vi "UI - Initiate Connection_second.vi"(8 "error in (no error)":errorcluster, 10 "Controller Address":string, 11 "Message Queue":refnum<queue>) -> (0 "error out":errorcluster, 1 "Connected?":bool)   [LabVIEW 2017]
uses:
  Message Queue/Message Cluster.ctl
  controls/FPGA State.ctl
  controls/CPU Loads.ctl
  <vilib>/vision/Image Controls.llb/IMAQ Image.ctl
  Globals/Global - Configuration Options.vi
  Globals/Global - UI Stream and Variable Connections.vi
  Message Queue/Message Queue.lvlib
panel:
  out "RT Stream Name":string="FanControlSampleProject_Command Stream from RT"
  out "UI Stream Name":string="FanControlSampleProject_Command Stream from UI"
  out "error out 4":errorcluster
  out "error out 3":errorcluster
  out "error out 2":errorcluster
  out "tag acc":refnum<k21>
  out "Tag acc":refnum<k21>
  out "Variable Name Control/Indicator 2":refnum<k21>
  out "Variable Name Control/Indicator":refnum<k21>
  out "resulting string 2":string
  out "reader name":string="UI Reader"
  out "writer name":string="UI Writer"
  out "resulting string":string
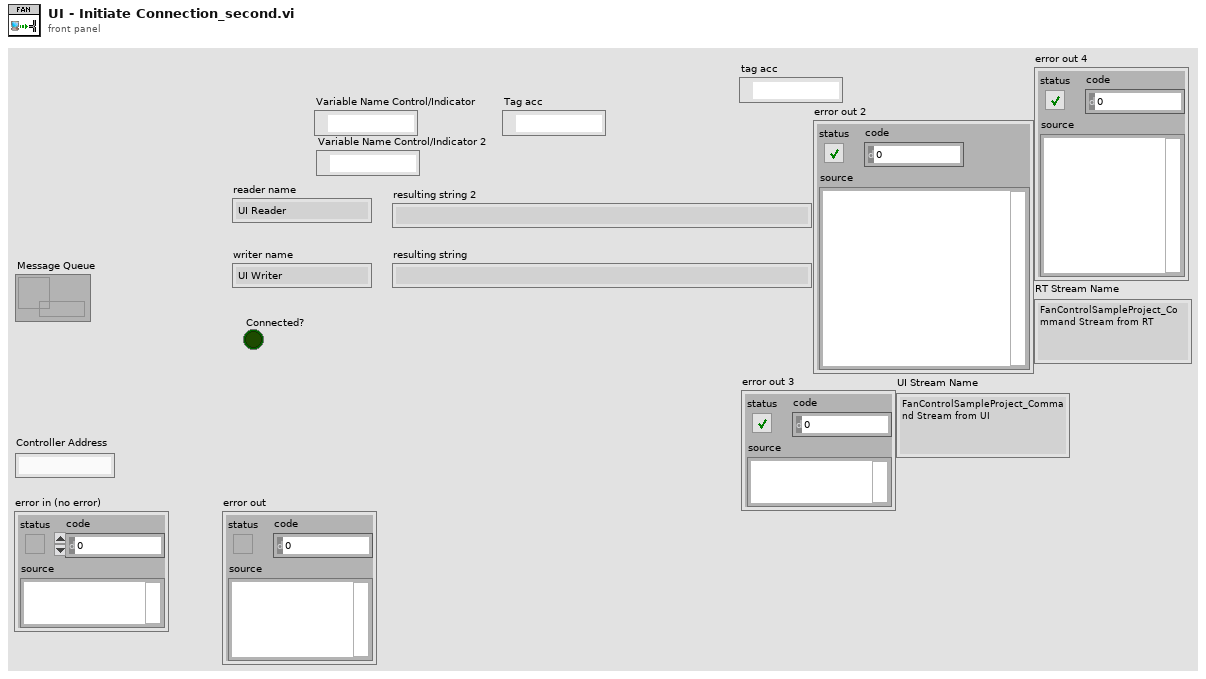
[diagram p1: front panel]
types:
  T1 = typedef "IMAQ Image.ctl" = refnum<image>
  T2 = typedef "CPU Loads.ctl" = cluster{"Total (%)":dbl, "Time Critical (%)":dbl, "Timed Structures (%)":dbl, "High (%)":dbl, "Above Normal (%)":dbl, "Normal (%)":dbl, "Background (%)":dbl, "Idle (%)":dbl, "ISR (%)":dbl}[]
  T3 = typedef "FPGA State.ctl" = enum16{"Safe State", "Control (PID)"}
  T4 = typedef "Message Queue.lvlib/Message Cluster.ctl" = cluster{"Message":string, "Message Data":variant}
  T5 = cluster{"Actual PID Loop Period":refnum<k21>, "DMA FIFO Overflow?":refnum<k21>, "CPU Usage":refnum<k21>, "Free or Contiguous Memory":refnum<k21>, "Current FPGA State":refnum<k21>, "Acceleration (grms)":refnum<k21>, "Acceleration Waveform":refnum<k21>, "Chatter":refnum<k21>, "tag acc":refnum<k21>, "tag video":refnum<k21>, "images":refnum<k21>}
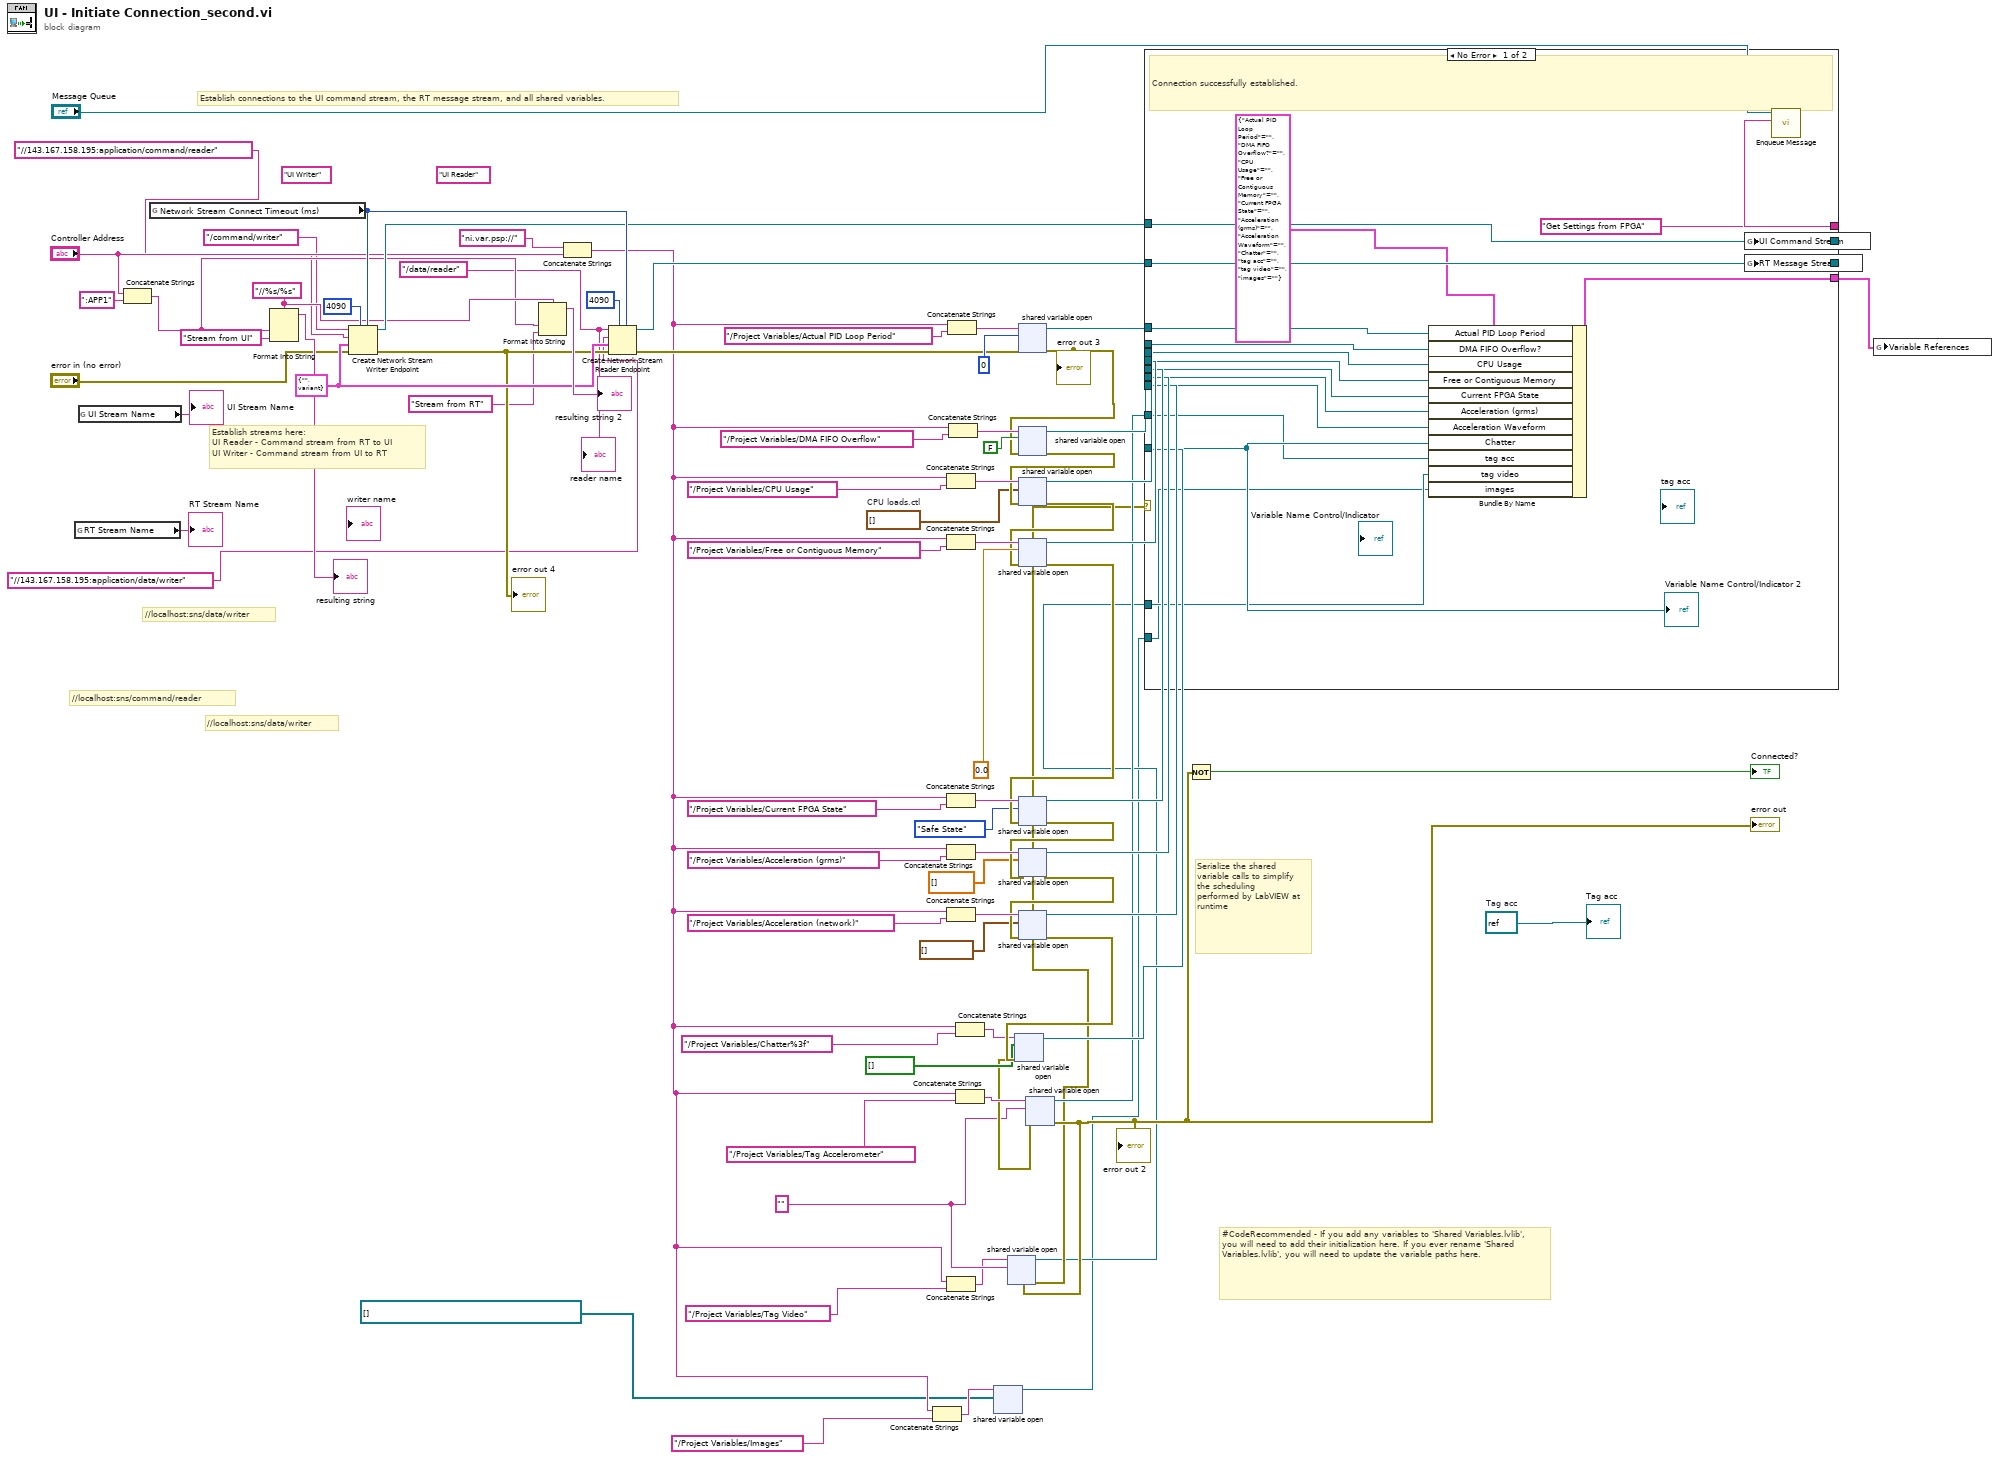
[diagram p0: block diagram]
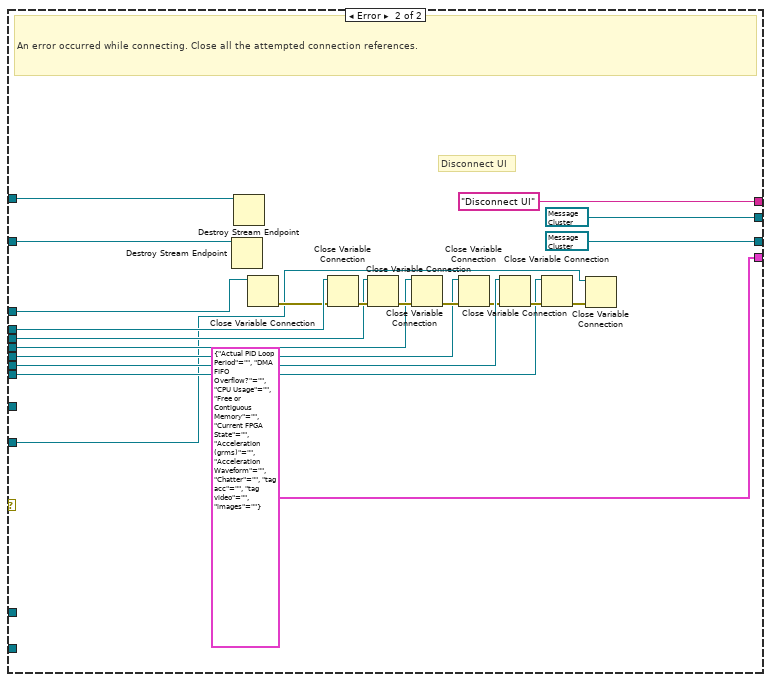
[diagram p2: hidden frame]
diagram:
  w2 = "/data/reader" ("writer name")
  (unwired) "UI Reader" ("reader name")
  w23 = "" ("string")
  w25 = refnum<k21> refnum  # Tag acc
  w38 = T2 []  # CPU loads.ctl
  w82 = T4 {"Message"="", "Message Data"=variant} ("Message Cluster")
  (unwired) "UI Writer" ("writer name")
  w30 = "//%s/%s"
  # "//localhost:sns/command/reader"
  # "//localhost:sns/data/writer"
  # "//localhost:sns/data/writer"
  # "Establish connections to the UI command stream, the RT message stream, and all shared variables."
  # "#CodeRecommended - If you add any variables to 'Shared Variables.lvlib', you will need to add their initialization here. If you ever rename 'Shared Variables.lvlib', you will need to update the variable paths here."
  # "Establish streams here:\nUI Reader - Command stream from RT to UI\nUI Writer - Command stream from UI to RT"
  # "Serialize the shared variable calls to simplify the scheduling performed by LabVIEW at runtime"
  n1 = global read "Global - Configuration Options.vi" "RT Stream Name"() -> (→"RT Stream Name":string)
  n2 = global read "Global - Configuration Options.vi" "UI Stream Name"() -> (→"UI Stream Name":string)
  n3 = Concatenate Strings("Controller Address", ":APP1" ("string")) -> (w9:string)
  n4 = global read "Global - Configuration Options.vi" "Network Stream Connect Timeout (ms)"() -> (w81:i32)
  n5 = Format Into String(format string=w30, w9, "Stream from UI" ("input 2")) -> (resulting string=→"resulting string":string)  [unwired: 2 in, 1 out]
  n6 = Create Network Stream Writer Endpoint(5:w81, 7:4090 ("writer buffer size"), 8:"error in (no error)", 9:w82, 10:"//143.167.158.195:application/command/reader" ("string"), 11:"/command/writer" ("writer name")) -> (0:w18:errorcluster, 3:w68:refnum<k21>)  [unwired: 1 in]
  "error out 4" <- w18
  n7 = Format Into String(format string=w30, w9, "Stream from RT" ("input 2")) -> (resulting string=→"resulting string 2":string)  [unwired: 2 in, 1 out]
  n8 = Concatenate Strings("ni.var.psp://", "Controller Address") -> (w15:string)
  n9 = Create Network Stream Reader Endpoint(5:w81, 7:4090 ("reader buffer size"), 8:w18, 9:w82, 10:"//143.167.158.195:application/data/writer" ("string"), 11:w2) -> (0:w61:errorcluster, 3:w67:refnum<k21>)  [unwired: 1 in]
  n10 = Concatenate Strings(w15, "/Project Variables/Images") -> (w17:string)
  n11 = Concatenate Strings(w15, "/Project Variables/CPU Usage") -> (w73:string)
  n12 = Concatenate Strings(w15, "/Project Variables/Free or Contiguous Memory") -> (w57:string)
  n13 = Concatenate Strings(w15, "/Project Variables/Current FPGA State") -> (w54:string)
  n14 = Concatenate Strings(w15, "/Project Variables/Acceleration (grms)") -> (w53:string)
  n15 = Concatenate Strings(w15, "/Project Variables/Acceleration (network)") -> (w50:string)
  n16 = Concatenate Strings(w15, "/Project Variables/Tag Video") -> (w19:string)
  n17 = Concatenate Strings(w15, "/Project Variables/Actual PID Loop Period") -> (w78:string)
  n18 = Concatenate Strings(w15, "/Project Variables/DMA FIFO Overflow") -> (w76:string)
  n19 = Concatenate Strings(w15, "/Project Variables/Chatter%3f") -> (w33:string)
  n20 = Concatenate Strings(w15, "/Project Variables/Tag Accelerometer") -> (w29:string)
  n21 = shared-variable-open(w17, T1[] []) -> (w13:refnum<k21>)  [unwired: 2 in, 1 out]
  n22 = shared-variable-open(w78, w61, u32 0) -> (w71:refnum<k21>, w31:errorcluster)  [unwired: 1 in]
  "error out 3" <- w31
  n23 = shared-variable-open(w76, w31, FALSE ("data type")) -> (w70:refnum<k21>, w72:errorcluster)  [unwired: 1 in]
  n24 = shared-variable-open(w73, w72, w38) -> (w69:refnum<k21>, w49:errorcluster)  [unwired: 1 in]
  n25 = shared-variable-open(w57, w49, 0.0) -> (w44:refnum<k21>, w48:errorcluster)  [unwired: 1 in]
  n26 = shared-variable-open(w54, w48, FPGA_State."Safe State" ("FPGA State")) -> (w43:refnum<k21>, w47:errorcluster)  [unwired: 1 in]
  n27 = shared-variable-open(w53, w47, dbl[] []) -> (w42:refnum<k21>, w46:errorcluster)  [unwired: 1 in]
  n28 = shared-variable-open(w50, w46, waveform(dbl)[] []) -> (w41:refnum<k21>, w35:errorcluster)  [unwired: 1 in]
  n29 = shared-variable-open(w33, w35, bool[] []) -> (w32:refnum<k21>, w26:errorcluster)  [unwired: 1 in]
  n30 = shared-variable-open(w29, w26, w23) -> (w27:refnum<k21>, w22:errorcluster)  [unwired: 1 in]
  "error out" <- w22
  "error out 2" <- w22
  n31 = shared-variable-open(w19, w22, w23) -> (w20:refnum<k21>, w21:errorcluster)  [unwired: 1 in]
  n32 = case shown="No Error" w21 {
    tunnel: w71 -> [w101 w119]
    tunnel: w70 -> [w97 w117]
    tunnel: w69 -> [w96 w118]
    tunnel: w68 -> [w98 w121]
    tunnel: w67 -> [w100 w122]
    tunnel: [w100 refnum<k21> refnum] -> w66
    tunnel: [w98 refnum<k21> refnum] -> w65
    tunnel: ["Get Settings from FPGA" "Disconnect UI"] -> w63
    tunnel: w44 -> [w95 w111]
    tunnel: w43 -> [w94 w110]
    tunnel: w42 -> [w93 w109]
    tunnel: w41 -> [w92 w106]
    tunnel: w32 -> [w91 w103]
    tunnel: w27 -> [w88 _]
    tunnel: [w89 T5 {"Actual PID Loop Period"="", "DMA FIFO Overflow?"="", "CPU Usage"="", "Free or Contiguous Memory"="", "Current FPGA State"="", "Acceleration (grms)"="", "Acceleration Waveform"="", "Chatter"="", "tag acc"="", "tag video"="", "images"=""} ("Variable References")] -> w12
    tunnel: w20 -> [w87 _]
    tunnel: w13 -> [w86 _]
    frame No Error {
      # "Connection successfully established."
      n33 = Bundle By Name(cluster=T5 {"Actual PID Loop Period"="", "DMA FIFO Overflow?"="", "CPU Usage"="", "Free or Contiguous Memory"="", "Current FPGA State"="", "Acceleration (grms)"="", "Acceleration Waveform"="", "Chatter"="", "tag acc"="", "tag video"="", "images"=""} ("Variable References"), "Actual PID Loop Period"=w101, "DMA FIFO Overflow?"=w97, "CPU Usage"=w96, "Free or Contiguous Memory"=w95, "Current FPGA State"=w94, "Acceleration (grms)"=w93, "Acceleration Waveform"=w92, "Chatter"=w91, "tag acc"=w88, "tag video"=w87, "images"=w86) -> (w89:T5)
      "Variable Name Control/Indicator 2" <- w91
    }
    frame Error {
      # "Disconnect UI"
      # "An error occurred while connecting. Close all the attempted connection references."
      n34 = Destroy Stream Endpoint(11:w122) -> ()  [unwired: 1 in, 1 out]
      n35 = Destroy Stream Endpoint(11:w121) -> ()  [unwired: 1 in, 1 out]
      n36 = Close Variable Connection(11:w119) -> (0:w105:errorcluster)  [unwired: 1 in]
      n37 = Close Variable Connection(8:w105, 11:w117) -> (0:w120:errorcluster)
      n38 = Close Variable Connection(8:w120, 11:w118) -> (0:w113:errorcluster)
      n39 = Close Variable Connection(8:w113, 11:w111) -> (0:w112:errorcluster)
      n40 = Close Variable Connection(8:w112, 11:w110) -> (0:w108:errorcluster)
      n41 = Close Variable Connection(8:w108, 11:w109) -> (0:w107:errorcluster)
      n42 = Close Variable Connection(8:w107, 11:w106) -> (0:w104:errorcluster)
      n43 = Close Variable Connection(8:w104, 11:w103) -> ()  [unwired: 1 out]
    }
  }
  n44 = Not(x=w22) -> (.not. x?=→"Connected?":bool)
  n45 = global write "Global - UI Stream and Variable Connections.vi" "UI Command Stream"(w65) -> ()
  n46 = global write "Global - UI Stream and Variable Connections.vi" "RT Message Stream"(w66) -> ()
  n47 = call "Enqueue Message.vi"("Message"=w63, "Message Queue"="Message Queue") -> ()  [unwired: 8 in, 2 out]
  n48 = global write "Global - UI Stream and Variable Connections.vi" "Variable References"(w12) -> ()
  "reader name" <- w2
  "Tag acc" <- w25
